vi "refraction_polarization_correction.vi"(8 "Error In":errorcluster) -> (0 "Error Out":errorcluster)   [LabVIEW 2019]
panel:
  in  "Refraction Polarization Correction Input":T1
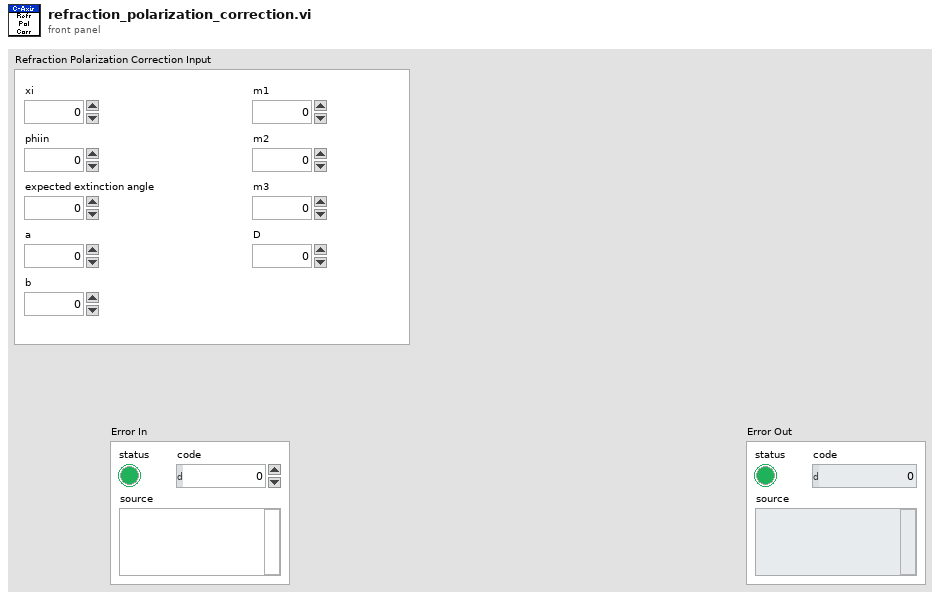
[diagram p1: front panel]
types:
  T1 = cluster{"xi":dbl, "phiin":dbl, "expected extinction angle":dbl, "a":dbl, "b":dbl, "m1":dbl, "m2":dbl, "m3":dbl, "D":dbl}
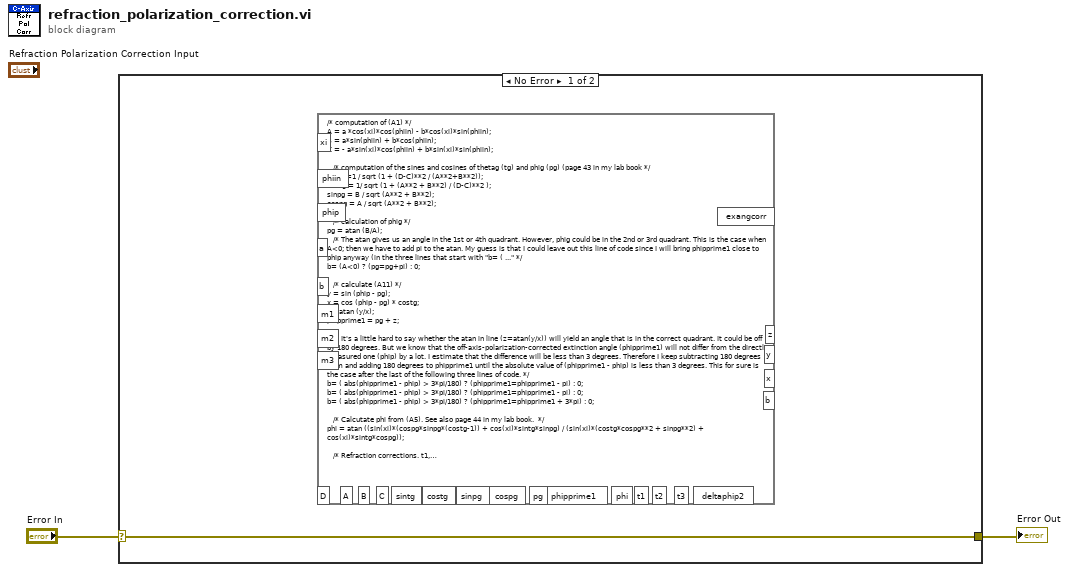
[diagram p0: block diagram]
diagram:
  n1 = case shown="No Error" "Error In" {
    selector: "Error In" -> [w3 w4]
    tunnel: [w3 w4] -> w1
    frame No Error {
      n2 = formula code="/* computation of (A1) */\nA = a *cos(xi)*cos(phiin) - b*cos(xi)*sin(phiin);\nB = a*sin(phiin) + b*cos(phiin);\nC = - a*sin(xi)*cos(phiin) + b*sin(xi)*sin(phiin);\n\n   /* computation of the sines and cosines of thetag (tg) and phig (pg) (page 43 in my lab book */\nsintg =1 / sqrt (1 + (D-C)**2 / (A**2+B**2));\ncostg = 1/ sqrt (1 + (A**2 + B**2) / (D-C)**2 );\nsinpg = B / sqrt (A**2 + B**2);\ncospg = A / sqrt (A**2 + B**2);\n\n   /* calculation of phig */\npg = atan (B/A);\n   /* The atan gives us an angle in the 1st or 4th quadrant. However, phig could be in the 2nd or 3rd quadrant. This is the case when A<0; then we have to add pi to the atan. My guess is that I could leave out this line of code since I will bring phipprime1 close to phip anyway (in the three lines that start with \"b= ( ...\" */\nb= (A<0) ? (pg=pg+pi) : 0;\n\n   /* calculate (A11) */\ny = sin (phip - pg);\nx = cos (phip - pg) * costg;\nz= atan (y/x);\nphipprime1 = pg + z;\n\n   /* It's a little hard to say whether the atan in line (z=atan(y/x)) will yield an angle that is in the correct quadrant. It could be off by 180 degrees. But we know that the off-axis-polarization-corrected extinction angle (phipprime1) will not differ from the directly measured one (phip) by a lot. I estimate that the difference will be less than 3 degrees. Therefore I keep subtracting 180 degrees from and adding 180 degrees to phipprime1 until the absolute value of (phipprime1 - phip) is less than 3 degrees. This for sure is the case after the last of the following three lines of code. */\nb= ( abs(phipprime1 - phip) > 3*pi/180) ? (phipprime1=phipprime1 - pi) : 0;\nb= ( abs(phipprime1 - phip) > 3*pi/180) ? (phipprime1=phipprime1 - pi) : 0;\nb= ( abs(phipprime1 - phip) > 3*pi/180) ? (phipprime1=phipprime1 + 3*pi) : 0;\n\n   /* Calcutate phi from (A5). See also page 44 in my lab book.  */\nphi = atan ((sin(xi)*(cospg*sinpg*(costg-1)) + cos(xi)*sintg*sinpg) / (sin(xi)*(costg*cospg**2 + sinpg**2) + cos(xi)*sintg*cospg));\n\n   /* Refraction corrections. t1, t2, and t3 stand for theta1, theta2, and theta3. (See page 49 of my lab book.) */ \nt1 = xi;\nt2 = asin (m1/m2 * sin (t1));\nt3 = asin (m1/m3 * sin (t1));\n\n   /* compute (A16) */\ndeltaphip2 = 0.5 * ( atan (tan (phip - phi) * cos (t1 - t2) * cos (t2 - t3)) - atan (tan(phip - phi) * cos (t3 - t1)));\n\n   /* Add the refraction correction to the off axis polarization corrected extinction angle. */ \nexangcorr = phipprime1 + deltaphip2;"() -> ()  [unwired: 9 in, 19 out]
    }
    frame Error {
    }
  }
  "Error Out" <- w1
